vi "Init Actor.vi"(9 "Name Specs":refnum<class "Name Specs.lvclass">, 10 "Project Stuff":refnum<class "Project Stuff.lvclass">) -> (3 "Actor out":refnum<class "Actor.lvclass">)   [LabVIEW 2020, in "_Rescript.lvlib" / "Actor.lvlib" / "Actor.lvclass"]
uses:
  Actor.lvclass
  _Shared/Project Stuff/Project Stuff.lvclass
  _Shared/Name Specs/Name Specs.lvclass
  Terminals.ctl
  Actor.lvclass/Actor.ctl
  _Rescript.lvlib
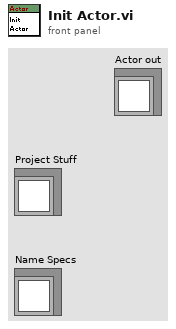
[diagram p1: front panel]
types:
  T1 = typedef "_Rescript.lvlib/Terminals.ctl" = set{i32}
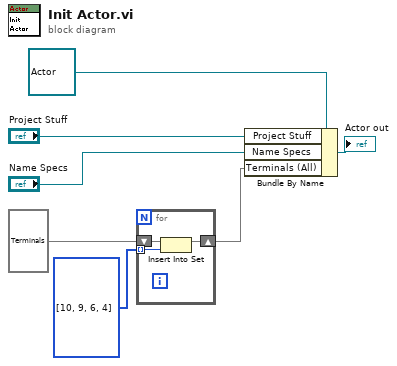
[diagram p0: block diagram]
diagram:
  n1 = for {
    tunnel: i32[] [10, 9, 6, 4] -> [w8] mode=indexing
    shift-right: [w9] -> w2
    shift-left: T1 {} ("All Terminals") -> [w10]
    n2 = Insert Into Set(10:w8, 11:w10) -> (3:w9:T1)  [unwired: 1 out]
  }
  n3 = Bundle By Name(cluster=refnum<class "Actor.lvclass"> refnum ("Actor out"), "Project Stuff"="Project Stuff", "Name Specs"="Name Specs", "Terminals (All)"=w2) -> (→"Actor out":refnum<class "Actor.lvclass">)
